vi "axis_DecodeData.vi"(8 "error IO":errorcluster, 9 "Data In":string, 11 "Image In":T1) -> (0 "error out":errorcluster={"status"=TRUE, "code"=-1074396120, "source"="IMAQ ReadFile\n  Not an image."}, 3 "Image Out":T1)   [LabVIEW 2012]
uses:
  <vilib>/vision/Image Controls.llb/IMAQ Image.ctl
  nivissvc.dll
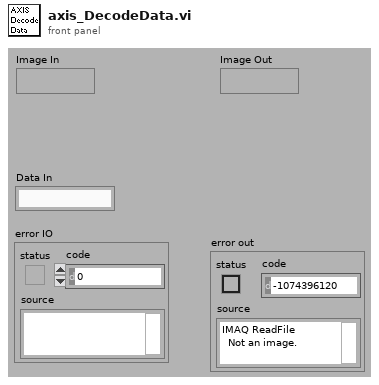
[diagram p1: front panel]
types:
  T1 = typedef "IMAQ Image.ctl" = refnum<image>
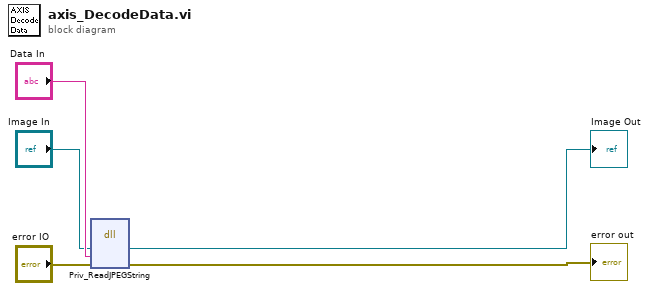
[diagram p0: block diagram]
diagram:
  n1 = dll-call lib="nivissvc.*" fn="Priv_ReadJPEGString"("Image"="Image In", "name"="Data In", "err"="error IO") -> ("Image"=→"Image Out":T1, "err"=→"error out":errorcluster)  [unwired: 4 in, 3 out]
